vi "Flatten Packets.vi"(10 "Incoming Packet":refnum<class "ControlPacket.lvclass">) -> (2 "Packets":refnum<class "ControlPacket.lvclass">[](array[class]))   [LabVIEW 2013, in "MQTT Server.lvlib" / "PacketCollection.lvclass"]
uses:
  PacketCollection.lvclass
  <vilib>/LabVIEW Open Source Project/MQTT Control Packets/Control Packets/ControlPacket/ControlPacket.lvclass
  PacketCollection.lvclass/PacketCollection.ctl
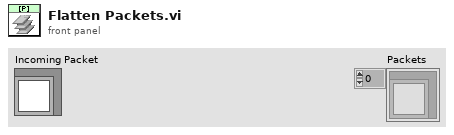
[diagram p1: front panel]
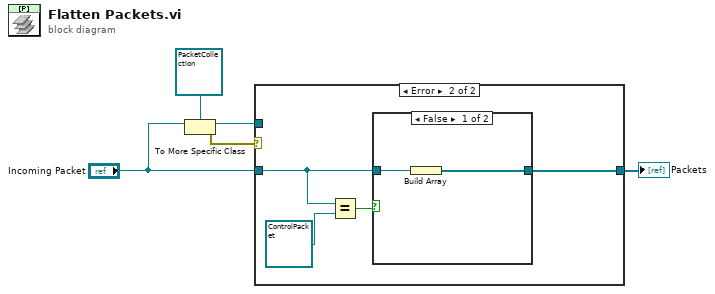
[diagram p0: block diagram]
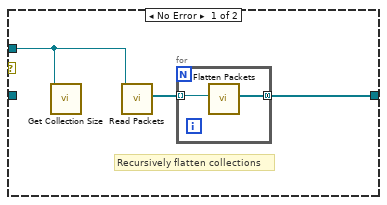
[diagram p2: hidden frame]
diagram:
  n1 = To More Specific Class(target class=refnum<class "PacketCollection.lvclass"> refnum ("PacketCollection in"), reference="Incoming Packet") -> (specific class reference=w3:refnum<class "PacketCollection.lvclass">, error out=w2:errorcluster)  [unwired: 1 in]
  n2 = case shown="Error" w2 {
    tunnel: [w8 w14] -> w5
    tunnel: w3 -> [w7 _]
    tunnel: "Incoming Packet" -> [_ w13]
    frame No Error {
      # "Recursively flatten collections"
      n3 = call "Get Collection Size.vi"("PacketCollection in"=w7) -> ()  [unwired: 9 in, 2 out]
      n4 = call "Read Packets.vi"("PacketCollection in"=w7) -> ("Packets"=w6:refnum<class "ControlPacket.lvclass">[])  [unwired: 9 in, 1 out]
      n5 = for {
        tunnel: w6 -> [w10] mode=indexing
        tunnel: [w9] -> w8 mode=concatenating
        n6 = call "Flatten Packets.vi"("Incoming Packet"=w10) -> ("Packets"=w9:refnum<class "ControlPacket.lvclass">[])  [unwired: 10 in]
      }
    }
    frame Error {
      n7 = Equal?(x=w13, y=refnum<class "ControlPacket.lvclass"> refnum) -> (x = y?=w11:bool)
      n8 = case shown="False" w11 {
        tunnel: [w16 _] -> w14
        tunnel: w13 -> [w15 _]
        frame False {
          n9 = Build Array(w15) -> (w16:refnum<class "ControlPacket.lvclass">[])
        }
        frame True {
        }
      }
    }
  }
  "Packets" <- w5
